vi "TEST.vi"() -> ()   [LabVIEW 2019]
uses:
  <vilib>/imath/engines/lvmath2/RunTimeEngine/Managers/WorkSpace/UID Generator.vi
  <vilib>/imath/engines/lvmath2/RunTimeEngine/RunTimeType/NIMS_RunTimeType_From StrictType (excl LVString).vi
  <instcachedir>/0/NIMS_RunTimeType_From StrictType (excl LVString)_D8AFBA86A94845AAA577C895450664BD.lvgen/NIMS_RunTimeType_From StrictType (excl LVString)_D8AFBA86A94845AAA577C895450664BD_000.vi
  <vilib>/imath/engines/lvmath2/RunTimeEngine/LocalVariableDefStatement/MC_LocalVariableDefStatement_Display.vi
  <vilib>/imath/engines/lvmath2/RunTimeEngine/BuiltInFunctions/diag/NIMS_diag.vi
  <instcachedir>/0/NIMS_diag_DCAB8C8FDAF64F9E84492BB524435AA9.lvgen/NIMS_diag_DCAB8C8FDAF64F9E84492BB524435AA9_003.vi
  <vilib>/imath/engines/lvmath2/RunTimeEngine/BuiltInFunctions/mirrorh/NIMS_mirrorh(GM).vi
  <instcachedir>/0/NIMS_mirrorh(GM)_A650AD0D730A4A8EBE251B4C5C7CA115.lvgen/NIMS_mirrorh(GM)_A650AD0D730A4A8EBE251B4C5C7CA115_004.vi
  <vilib>/imath/engines/lvmath2/RunTimeEngine/RowToken/NIMS_RowToken_M_M.vi
  <instcachedir>/0/NIMS_RowToken_M_M_21FE36D058524603B8B587AC30FD72C2.lvgen/NIMS_RowToken_M_M_21FE36D058524603B8B587AC30FD72C2_005.vi
  <vilib>/imath/engines/lvmath2/RunTimeEngine/ErrorHandling/NIMS_Create Error From Enums.vi
  <vilib>/imath/engines/lvmath2/RunTimeEngine/Managers/SymbolTable/Clear UID.vi
  <vilib>/imath/engines/lvmath2/RunTimeEngine/NodeEndStatement/NIMS_NodeEndStatement_Output.vi
  <instcachedir>/0/NIMS_NodeEndStatement_Output_53EC0D466D134D7ABD903AC30B43404B.lvgen/NIMS_NodeEndStatement_Output_53EC0D466D134D7ABD903AC30B43404B_005.vi
  <instcachedir>/0/NIMS_NodeEndStatement_Output_53EC0D466D134D7ABD903AC30B43404B.lvgen/NIMS_NodeEndStatement_Output_53EC0D466D134D7ABD903AC30B43404B_002.vi
  <instcachedir>/0/NIMS_NodeEndStatement_Output_53EC0D466D134D7ABD903AC30B43404B.lvgen/NIMS_NodeEndStatement_Output_53EC0D466D134D7ABD903AC30B43404B_010.vi
  <vilib>/imath/engines/lvmath2/RunTimeEngine/ErrorHandling/NIMS_Finalize Error.vi
  OneDrive/Documents/LabVIEW Data/MathScriptVIs/MCStatic_41946317732_39d282e6f644b4de5e03d5ec5e14f762.vi
  <instcachedir>/0/MCStatic_41946317732_39d282e6f644b4de5e03d5ec5e14f762_F82D6288F92F4DD7BE24A1113A5A915E.lvgen/MCStatic_41946317732_39d282e6f644b4de5e03d5ec5e14f762_F82D6288F92F4DD7BE24A1113A5A915E_000.vi
  <vilib>/imath/engines/lvmath2/RunTimeEngine/ArithmeticOperatorToken/NIMS_ArithmeticOperator_multmx.vi
  <instcachedir>/0/NIMS_ArithmeticOperator_multmx_77F1D2D6F4D94BA7A97C4E7185C02392.lvgen/NIMS_ArithmeticOperator_multmx_77F1D2D6F4D94BA7A97C4E7185C02392_003.vi
  <vilib>/imath/engines/lvmath2/RunTimeEngine/BuiltInFunctions/inv/NIMS_inv(GM).vi
  <instcachedir>/0/NIMS_inv(GM)_A6DF8FE880224208AACFE4CF9F659502.lvgen/NIMS_inv(GM)_A6DF8FE880224208AACFE4CF9F659502_001.vi
  Analytic_Jacobian_Mag_cir_array_noM.m
  <vilib>/imath/engines/lvmath2/RunTimeEngine/Managers/SymbolTable/NIMS_WorkSpace.lvlib
panel:
  out "TIme":u32
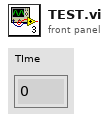
[diagram p1: front panel]
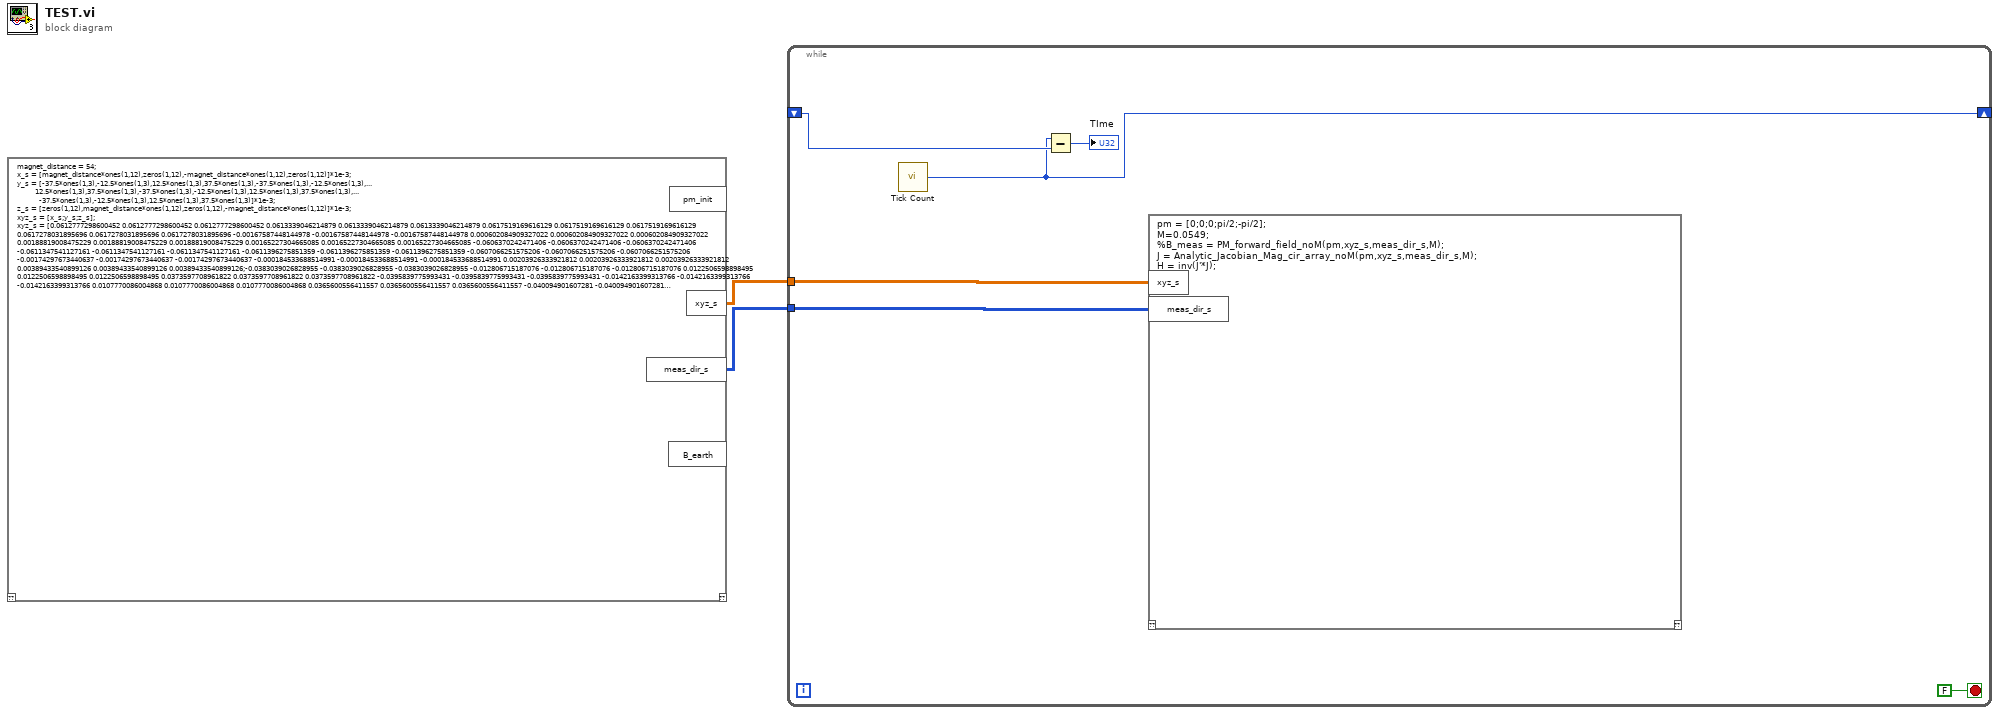
[diagram p0: block diagram]
diagram:
  n1 = mathscript code="magnet_distance = 54;\nx_s = [magnet_distance*ones(1,12),zeros(1,12),-magnet_distance*ones(1,12),zeros(1,12)]*1e-3; \ny_s = [-37.5*ones(1,3),-12.5*ones(1,3),12.5*ones(1,3),37.5*ones(1,3),-37.5*ones(1,3),-12.5*ones(1,3),...\n         12.5*ones(1,3),37.5*ones(1,3),-37.5*ones(1,3),-12.5*ones(1,3),12.5*ones(1,3),37.5*ones(1,3),...\n           -37.5*ones(1,3),-12.5*ones(1,3),12.5*ones(1,3),37.5*ones(1,3)]*1e-3; \nz_s = [zeros(1,12),magnet_distance*ones(1,12),zeros(1,12),-magnet_distance*ones(1,12)]*1e-3; \nxyz_s = [x_s;y_s;z_s];  \nxyz_s = [0.0612777298600452 0.0612777298600452 0.0612777298600452 0.0613339046214879 0.0613339046214879 0.0613339046214879 0.0617519169616129 0.0617519169616129 0.0617519169616129 0.0617278031895696 0.0617278031895696 0.0617278031895696 -0.00167587448144978 -0.00167587448144978 -0.00167587448144978 0.000602084909327022 0.000602084909327022 0.000602084909327022 0.00188819008475229 0.00188819008475229 0.00188819008475229 0.00165227304665085 0.00165227304665085 0.00165227304665085 -0.0606370242471406 -0.0606370242471406 -0.0606370242471406 -0.0611347541127161 -0.0611347541127161 -0.0611347541127161 -0.0611396275851359 -0.0611396275851359 -0.0611396275851359 -0.0607066251575206 -0.0607066251575206 -0.0607066251575206 -0.00174297673440637 -0.00174297673440637 -0.00174297673440637 -0.000184533688514991 -0.000184533688514991 -0.000184533688514991 0.00203926333921812 0.00203926333921812 0.00203926333921812 0.00389433540899126 0.00389433540899126 0.00389433540899126;-0.0383039026828955 -0.0383039026828955 -0.0383039026828955 -0.012806715187076 -0.012806715187076 -0.012806715187076 0.0122506598898495 0.0122506598898495 0.0122506598898495 0.0373597708961822 0.0373597708961822 0.0373597708961822 -0.0395839775993431 -0.0395839775993431 -0.0395839775993431 -0.0142163399313766 -0.0142163399313766 -0.0142163399313766 0.0107770086004868 0.0107770086004868 0.0107770086004868 0.0365600556411557 0.0365600556411557 0.0365600556411557 -0.040094901607281 -0.040094901607281 -0.040094901607281 -0.0149090266343068 -0.0149090266343068 -0.0149090266343068 0.0107078118967093 0.0107078118967093 0.0107078118967093 0.0356978973873521 0.0356978973873521 0.0356978973873521 -0.0392056799428433 -0.0392056799428433 -0.0392056799428433 -0.0139322320487061 -0.0139322320487061 -0.0139322320487061 0.0112429513248133 0.0112429513248133 0.0112429513248133 0.0361205812401305 0.0361205812401305 0.0361205812401305;0.00307213814961651 0.00307213814961651 0.00307213814961651 0.0033242461093476 0.0033242461093476 0.0033242461093476 0.00389293419390068 0.00389293419390068 0.00389293419390068 0.00390199978115286 0.00390199978115286 0.00390199978115286 0.0640688323293379 0.0640688323293379 0.0640688323293379 0.0636929900573754 0.0636929900573754 0.0636929900573754 0.0635181326061399 0.0635181326061399 0.0635181326061399 0.0633759954094267 0.0633759954094267 0.0633759954094267 -0.00381527257187291 -0.00381527257187291 -0.00381527257187291 -0.00312975643341264 -0.00312975643341264 -0.00312975643341264 -0.00272771938684928 -0.00272771938684928 -0.00272771938684928 -0.00268843620404175 -0.00268843620404175 -0.00268843620404175 -0.0628805002941716 -0.0628805002941716 -0.0628805002941716 -0.063138590462401 -0.063138590462401 -0.063138590462401 -0.063695098330538 -0.063695098330538 -0.063695098330538 -0.0638823957044235 -0.0638823957044235 -0.0638823957044235]\nmeas_dir_s = [mirrorh(diag([1;-1;1])),...\n              mirrorh(diag([1;-1;1])),...\n              mirrorh(diag([1;-1;1])),...\n              mirrorh(diag([1;-1;1])),...\n              diag([-1;-1;1]),...\n              diag([-1;-1;1]),...\n              diag([-1;-1;1]),...\n              diag([-1;-1;1]),...\n              mirrorh(diag([-1;-1;-1])),...\n              mirrorh(diag([-1;-1;-1])),...\n              mirrorh(diag([-1;-1;-1])),...\n              mirrorh(diag([-1;-1;-1])),... \n              diag([1;-1;-1]),...\n              diag([1;-1;-1]),...\n              diag([1;-1;-1]),...\n              diag([1;-1;-1])];\npm_init = [0;0;0;pi/2;-pi/2];\nB_earth = [-0.553111111\t-0.374555556\t-0.122619048...\n-0.515809524\t-0.295809524\t-0.077047619...\n-0.636904762\t-0.354634921\t-0.125174603...\n-0.544126984\t-0.318142857\t-0.118666667...\n0.235396825\t-0.012873016\t-0.451079365...\n0.087587302\t-0.320460317\t-0.478063492...\n0.075079365\t-0.297063492\t-0.457571429...\n0.078126984\t-0.341047619\t-0.499793651...\n0.401380952\t-0.248206349\t0.061952381...\n0.469435484\t-0.180274194\t0.06766129...\n0.442419355\t-0.269870968\t0.077758065...\n0.489177419\t-0.270806452\t-0.108483871...\n0.009730159\t-0.086761905\t0.67131746...\n-0.059096774\t-0.115145161\t0.576403226...\n-0.076854839\t-0.088258065\t0.584709677...\n-0.100354839\t-0.071241935\t0.519322581]';\nB_earth = [-0.567333\t\t-0.364333\t\t-0.155...\n-0.535667\t-0.278667\t\t-0.131...\n-0.669\t\t-0.355333\t\t-0.165...\n-0.562\t\t-0.300667\t\t-0.163667...\n0.278333\t-0.006\t\t-0.464333...\n0.126667\t-0.311\t\t-0.51...\n0.117667\t-0.29\t\t-0.499333...\n0.116\t\t-0.326667\t\t-0.534333...\n0.468667\t-0.243667\t\t0.04...\n0.506667\t-0.171667\t\t0.116...\n0.476\t\t-0.279333\t\t0.0543333...\n0.538667\t-0.255\t\t-0.0236667...\n-0.0566667\t-0.0843333\t\t0.678667...\n-0.126667\t-0.107667\t\t0.598333...\n-0.147333\t-0.0766667\t\t0.605...\n-0.172333\t-0.0466667\t\t0.542]';"() -> ("meas_dir_s"=w2:i32[][], "xyz_s"=w1:dbl[][])  [unwired: 1 in, 3 out]
  n2 = while {
    tunnel: w2 -> [w7]
    tunnel: w1 -> [w6]
    shift-right: [w4] -> _
    shift-left: _ -> [w5]
    stop <- FALSE stop-if-true
    n3 = call "Tick Count"() -> ("Tick Count(uSec)"=w4:u32)
    n4 = Subtract(x=w4, y=w5) -> (x-y=→"TIme":u32)
    n5 = mathscript code="pm = [0;0;0;pi/2;-pi/2]; \nM=0.0549;\n%B_meas = PM_forward_field_noM(pm,xyz_s,meas_dir_s,M);\nJ = Analytic_Jacobian_Mag_cir_array_noM(pm,xyz_s,meas_dir_s,M);\nH = inv(J'*J);"("xyz_s"=w6, "meas_dir_s"=w7) -> ()  [unwired: 1 in, 1 out]
  }
